vi "Tektronix_Enable_Channel_Mode.vi"(4 "Trigger Mode (0: Auto)":i32(ring) items=["Auto", "Normal"], 5 "等待时间（毫秒）":u32, 6 "error in (no error)":errorcluster, 7 "TestIndex":i32, 8 "Enable Channel":bool, 9 "Oscilloscope-Change":bool=TRUE, 10 "Channel (0: Channel 1)":i32(ring) items=["Channel 1", "Channel 2", "Channel 3", "Channel 4"]) -> (0 "error out":errorcluster, 3 "VISA":refnum<visa-resource-name>)   [LabVIEW 2015]
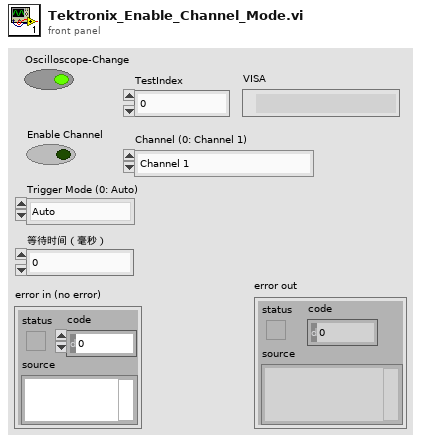
[diagram p1: front panel]
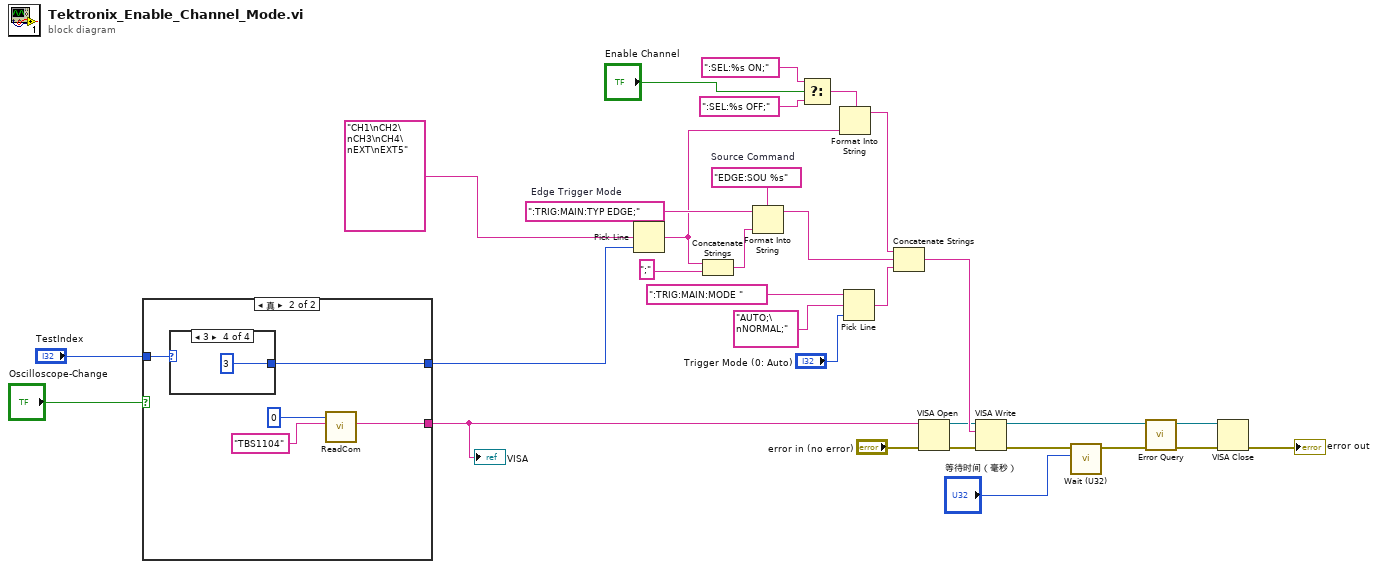
[diagram p0: block diagram]
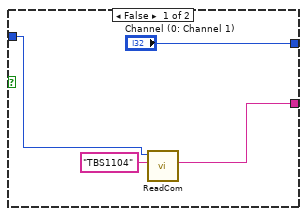
[diagram p2: hidden frame]
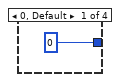
[diagram p3: hidden frame]
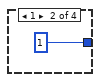
[diagram p4: hidden frame]
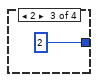
[diagram p5: hidden frame]
diagram:
  w25 = "EDGE:SOU %s"  # Source Command
  w27 = ":TRIG:MAIN:TYP EDGE;"  # Edge Trigger Mode
  n1 = case shown="真" "Oscilloscope-Change" {
    tunnel: ["Channel (0: Channel 1)" w40] -> w26
    tunnel: "TestIndex" -> [w32 w39]
    tunnel: [w34 w37] -> w1
    frame False {
      n2 = call "ReadCom.vi"("仪器名称"="TBS1104", "MyIndex"=w32) -> ("COM"=w34:string)  [unwired: 7 in, 2 out]
    }
    frame True {
      n3 = case shown="3" w39 {
        tunnel: [0 1 2 3] -> w40
        frame 0, Default {
        }
        frame 1 {
        }
        frame 2 {
        }
        frame 3 {
        }
      }
      n4 = call "ReadCom.vi"("仪器名称"="TBS1104", "MyIndex"=u8 0) -> ("COM"=w37:string)  [unwired: 7 in, 2 out]
    }
  }
  "VISA" <- w1
  n5 = Pick Line(multi-line string="CH1\nCH2\nCH3\nCH4\nEXT\nEXT5", line index=w26) -> (output string=w17:string)  [unwired: 1 out]
  n6 = Concatenate Strings(w17, ";") -> (w16:string)
  n7 = Format Into String(format string=w25, initial string=w27, w16) -> (resulting string=w21:string)  [unwired: 1 in, 1 out]
  n8 = Select(t=":SEL:%s ON;" ("format string"), s="Enable Channel", f=":SEL:%s OFF;" ("format string")) -> (s? t:f=w20:string)
  n9 = Format Into String(format string=w20, w17) -> (resulting string=w15:string)  [unwired: 2 in, 1 out]
  n10 = Pick Line(string ("")=":TRIG:MAIN:MODE ", multi-line string="AUTO;\nNORMAL;", line index="Trigger Mode (0: Auto)") -> (output string=w14:string)
  n11 = Concatenate Strings(w15, w21, w14) -> (w13:string)
  n12 = VISA Open(error in (no error)="error in (no error)", VISA resource name=w1) -> (VISA resource name=w9:refnum<visa-resource-name>, error out=w8:errorcluster)  [unwired: 3 in]
  n13 = VISA Write(VISA resource name=w9, write buffer=w13, error in (no error)=w8) -> (VISA resource name out=w31:refnum<visa-resource-name>, error out=w4:errorcluster)  [unwired: 1 out]
  n14 = call "Wait (U32).vi"("ms"="等待时间（毫秒）", "Error In"=w4) -> ("Error Out"=w3:errorcluster)  [unwired: 5 in]
  n15 = call "Error Query.vi"("error in (no error)"=w3, "VISA resource name"=w31) -> ("error out"=w12:errorcluster, "VISA resource name out"=w10:refnum<visa-resource-name>)  [unwired: 8 out]
  n16 = VISA Close(VISA resource name=w10, error in (no error)=w12) -> (error out=→"error out":errorcluster)
